vi "Analog Input Voltages.vi"(8 "error in (no error)":errorcluster, 10 "Analog Input Voltages":waveform(dbl)[](array[waveform]), 11 "Analog Input Interface Messages in":refnum<class "Analog Input Interface Messages.lvclass">) -> (0 "error out":errorcluster, 3 "Analog Input Interface Messages out":refnum<class "Analog Input Interface Messages.lvclass">)   [LabVIEW 2021, in "Analog Input Interface Messages.lvlib" / "Analog Input Interface Messages.lvclass"]
uses:
  Analog Input Interface Messages.lvclass
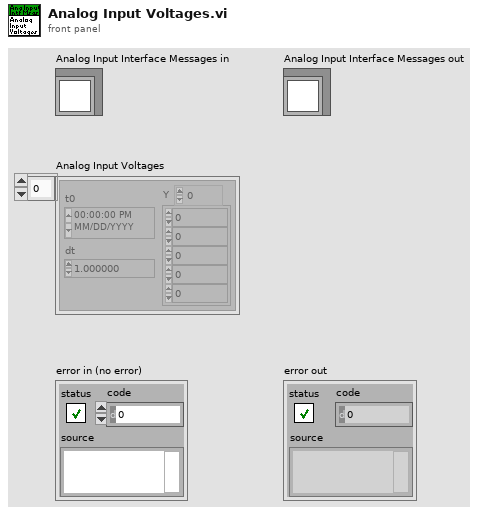
[diagram p1: front panel]
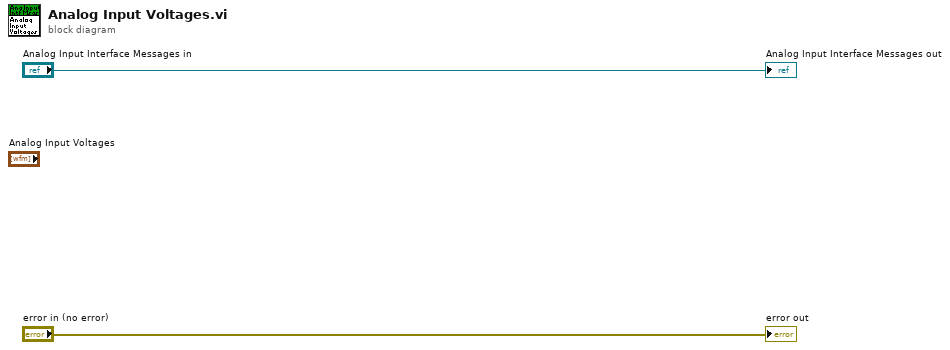
[diagram p0: block diagram]
diagram:
  "error out" <- "error in (no error)"
  "Analog Input Interface Messages out" <- "Analog Input Interface Messages in"
